vi "sub build i data.vi"(8 "error in":errorcluster, 11 "<i> data":T1) -> (0 "error out":errorcluster, 3 "<i> string":string)   [LabVIEW 2018, in "Data Parser.lvclass"]
uses:
  Data Parser.lvclass
  frame i data.ctl
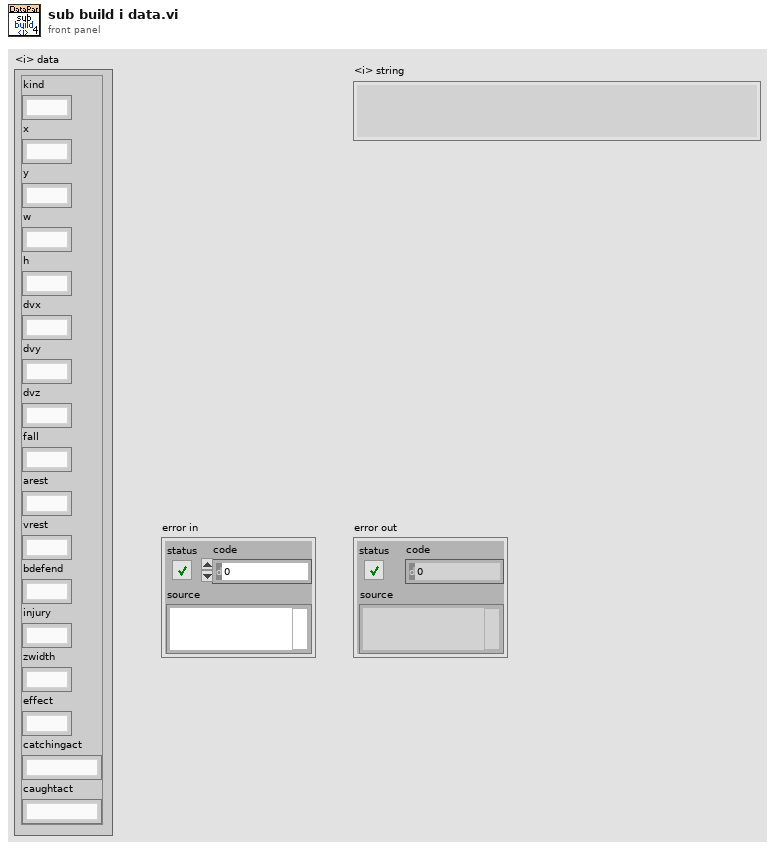
[diagram p1: front panel]
types:
  T1 = typedef "Data Parser.lvclass/frame i data.ctl" = cluster{"kind":string, "x":string, "y":string, "w":string, "h":string, "dvx":string, "dvy":string, "dvz":string, "fall":string, "arest":string, "vrest":string, "bdefend":string, "injury":string, "zwidth":string, "effect":string, "catchingact":string, "caughtact":string}
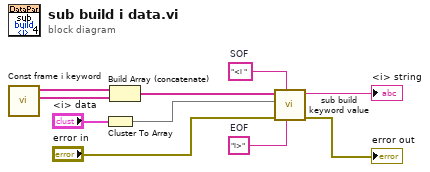
[diagram p0: block diagram]
diagram:
  w6 = "<i "  # SOF
  w4 = "i>"  # EOF
  n1 = call "Const frame i keyword.vi"() -> ("Const frame i keyword 2"=w2:string[], "Const frame i keyword"=w3:string[])  [unwired: 10 in]
  n2 = Cluster To Array(cluster="<i> data") -> (array=w5:string[])
  n3 = Build Array (concatenate)(w3, w2) -> (w1:string[])
  n4 = call "sub build keyword value.vi"("EOF"=w4, "SOF"=w6, "error in"="error in", "value"=w5, "keyword"=w1) -> ("error out"=→"error out":errorcluster, "keyword value string"=→"<i> string":string)  [unwired: 5 in]
